vi "CAN发车速.vi"() -> ()   [LabVIEW 2020]
uses:
  ZLG_CAN.lvlib
panel:
  in  "周期(ms)":u32=10 min=1 format="%d ms"
  in  "帧格式":enum16{"数据帧", "远程帧"}(ring)
  in  "帧类型":enum8{"标准帧", "扩展帧"}(ring)
  in  "ID":u32 format="0x%x"
  in  "波特率":u32(ring)=11 items=["5Kbps", "10Kbps", "20Kbps", "40Kbps", "50Kbps", "80Kbps", "100Kbps", "125Kbps", "200Kbps", "250Kbps", "400Kbps", "500Kbps", "666Kbps", "800Kbps", "1000Kbps"]
  in  "CAN 通道":u32(ring) items=["0", "1"]
  in  "索引":u32(ring) items=["0", "1", "2", "3", "4", "5", "6", "7", "8"]
  in  "设备类型":u32(ring)=3 items=["PCI5121"=1, "PCI9810"=2, "USBCAN1"=3, "USBCAN2"=4, "PCI9820"=5, "PCI5110"=7, "PC104CAN"=11, "CANETUDP"=12, "PCI9840B"=14, "PC104C2"=15, "PCI9820I"=16, "CANETTCP"=17, "PCIE9221"=24, "PCI5010U"=19, "USBCAN_E_U"=20, "USBCAN_2E_U"=21, "PCI5020U"=22, "PCIE9120I"=27, "PCIE9110I"=28, "PCIE9140I"=29]
  in  "Stop":bool
  # "Data Read"
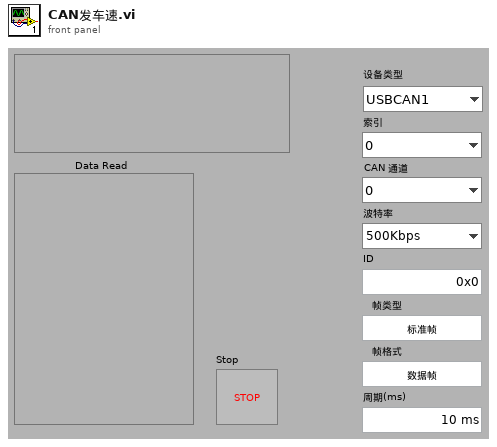
[diagram p1: front panel]
types:
  T1 = typedef "ZLG_CAN.lvlib/Start_CAN (Reply Payload)--cluster.ctl" = cluster{"Success":bool, "Start_CAN_error":errorcluster}
  T2 = cluster{u8, u8, "y":u8, "y":u8, "y":u8, "y":u8, "y":u8, "y":u8}
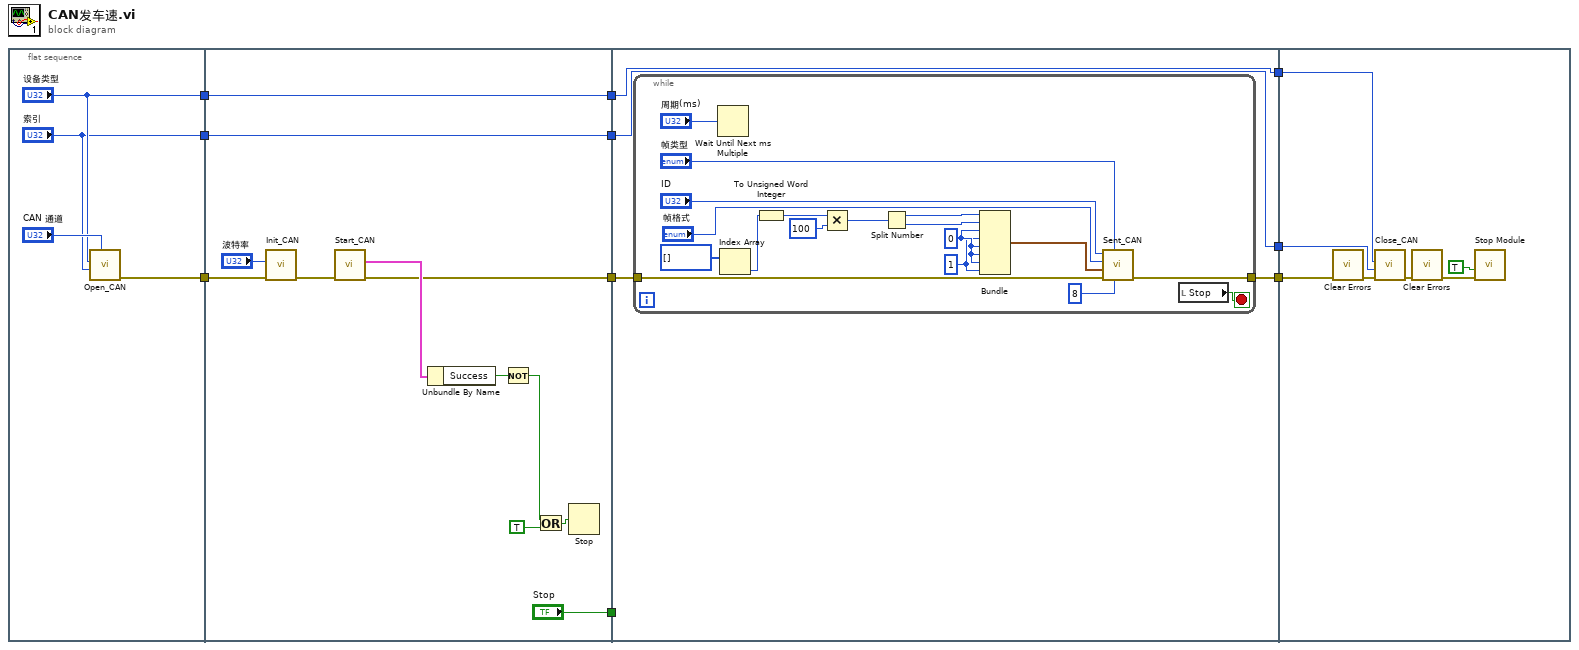
[diagram p0: block diagram]
diagram:
  n1 = flat-sequence {
    tunnel: ["索引"] -> w4
    tunnel: ["设备类型"] -> w3
    tunnel: [w12] -> w2
    tunnel: [w25] -> w10
    tunnel: [w20] -> w8
    tunnel: [w21] -> w6
    tunnel: w4 -> [w21]
    tunnel: w3 -> [w20]
    tunnel: w2 -> [w19]
    tunnel: ["Stop"] -> w1
    tunnel: w10 -> [w30]
    tunnel: [w29] -> w9
    tunnel: w8 -> [w28]
    tunnel: [w28] -> w7
    tunnel: w6 -> [w27]
    tunnel: [w27] -> w5
    tunnel: w1 -> [_]
    tunnel: w9 -> [w55]
    tunnel: w7 -> [w54]
    tunnel: w5 -> [w53]
    frame #0 {
      n2 = call "Open_CAN.vi"("CAN 通道"="CAN 通道", "索引"="索引", "设备类型"="设备类型") -> ("error out"=w12:errorcluster)  [unwired: 8 in]
    }
    frame #1 {
      n3 = call "Init_CAN.vi"("error in (no error)"=w19, "波特率"="波特率") -> ("error out"=w22:errorcluster)  [unwired: 9 in]
      n4 = call "Start_CAN.vi"("error in (no error)"=w22) -> ("error out"=w25:errorcluster, "Reply Payload"=w26:T1)  [unwired: 8 in, 1 out]
      n5 = Unbundle By Name(w26) -> ("Success"=w24:bool)
      n6 = Not(x=w24) -> (.not. x?=w17:bool)
      n7 = Or(x=w17, y=TRUE) -> (x .or. y?=w23:bool)
      n8 = Stop(stop? (T)=w23) -> ()
    }
    frame #2 {
      n9 = while {
        tunnel: w30 -> [w48]
        tunnel: [w46] -> w29
        stop <- w47 stop-if-true
        w38 = u8 1 ("y")
        w39 = u8 0 ("y")
        n10 = Wait Until Next ms Multiple(millisecond multiple="周期(ms)") -> ()  [unwired: 1 out]
        n11 = Index Array(array=u8[] [] ("数组")) -> (element=w45:u8)  [unwired: 1 in]
        n12 = To Unsigned Word Integer(number=w45) -> (unsigned 16bit integer=w43:u16)
        n13 = Multiply(x=w43, y=u16 100) -> (x*y=w42:u16)
        n14 = Split Number(x=w42) -> (hi(x)=w41:u8, lo(x)=w40:u8)
        n15 = Bundle(w41, w40, "y"=w39, "y"=w38, "y"=w39, "y"=w39, "y"=w39, "y"=w38) -> (w37:T2)  [unwired: 1 in]
        n16 = call "Sent_CAN.vi"("帧长度"=u8 8, "帧类型"="帧类型", "error in (no error)"=w48, "帧数据"=w37, "帧格式"="帧格式", "ID"="ID") -> ("error out"=w46:errorcluster)  [unwired: 5 in]
        n17 = local read "Stop"() -> (w47:bool)
      }
    }
    frame #3 {
      n18 = call <vilib>:"Clear Errors.vi"("error in (no error)"=w55) -> ("error out"=w49:errorcluster)  [unwired: 5 in, 1 out]
      n19 = call "Close_CAN.vi"("error in (no error)"=w49, "索引"=w53, "设备类型"=w54) -> ("error out"=w52:errorcluster)  [unwired: 8 in]
      n20 = call <vilib>:"Clear Errors.vi"("error in (no error)"=w52) -> ("error out"=w50:errorcluster)  [unwired: 5 in, 1 out]
      n21 = call "Stop Module.vi"("error in (no error)"=w50, "Wait for Module to Stop? (F)"=TRUE) -> ()  [unwired: 9 in, 1 out]
    }
  }
